vi "Get ID Number.vi"() -> (2 "id number":u32)   [LabVIEW 2018, in "Board Design.lvclass"]
doc: "Get an identification number."
uses:
  Board Design.lvclass
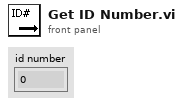
[diagram p1: front panel]
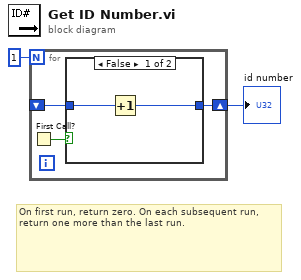
[diagram p0: block diagram]
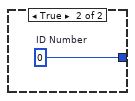
[diagram p2: hidden frame]
diagram:
  # "On first run, return zero. On each subsequent run, return one more than the last run."
  n1 = for {
    N: 1 -> [_]
    shift-right: [w4] -> w1
    shift-left: _ -> [w3]
    n2 = First Call?() -> (First Call?: T/F=w5:bool)
    n3 = case shown="False" w5 {
      tunnel: [w6 w8] -> w4
      tunnel: w3 -> [w7 _]
      frame False {
        n4 = Increment(x=w7) -> (x+1=w6:u32)
      }
      frame True {
        w8 = u32 0  # ID Number
      }
    }
  }
  "id number" <- w1
